vi "InitializeTC01.vi"(8 "error in":errorcluster, 10 "physical channel":string="Dev2/ai0", 11 "thermocouple type":i32(ring)=10072 items=["J"=10072, "K"=10073, "N"=10077, "R"=10082, "S"=10085, "T"=10086, "B"=10047, "E"=10055]) -> (0 "error out":errorcluster, 3 "task out":refnum<k21>)   [LabVIEW 2012]
uses:
  <vilib>/DAQmx/create/channels.llb/DAQmx Create Channel (AI-Temperature-Thermocouple).vi
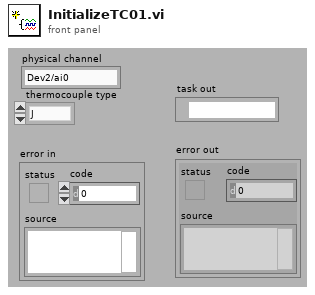
[diagram p1: front panel]
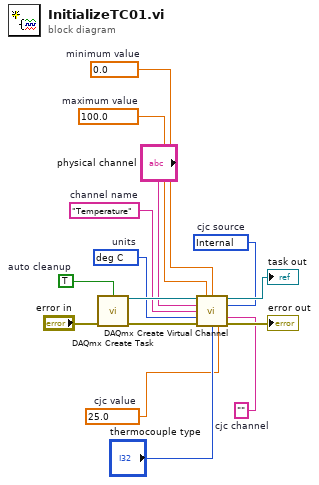
[diagram p0: block diagram]
diagram:
  w2 = ""  # cjc channel
  w3 = u32 10200 items=["Internal"=10200, "Constant Value"=10116, "Channel"=10113]  # cjc source
  w4 = 25.0  # cjc value
  w6 = 10143 items=["deg C"=10143, "deg F"=10144, "Kelvins"=10325, "deg R"=10145, "From Custom Scale"=10065]  # units
  w1 = "Temperature"  # channel name
  w9 = 0.0  # minimum value
  w10 = 100.0  # maximum value
  w13 = TRUE  # auto cleanup
  n1 = call <vilib>:"DAQmx Create Task.vi"("auto cleanup"=w13, "error in"="error in") -> ("task out"=w12:refnum<k21>, "error out"=w14:errorcluster)  [unwired: 3 in, 9 out]
  n2 = call-poly <vilib>:"DAQmx Create Virtual Channel.vi"("task in"=w12, "maximum value"=w10, "minimum value"=w9, "physical channels"="physical channel", "cjc source"=w3, "name to assign"=w1, "units"=w6, "cjc channel"=w2, "error in"=w14, "thermocouple type"="thermocouple type", "cjc value"=w4) -> ("task out"=→"task out":refnum<k21>, "error out"=→"error out":errorcluster)  [unwired: 2 in, 1 out]
